vi "MKS test.vi"() -> ()   [LabVIEW 2022 SP3]
uses:
  MKS.lvclass
panel:
  out "Data":dbl[](array[numeric])
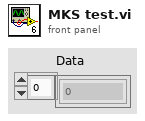
[diagram p1: front panel]
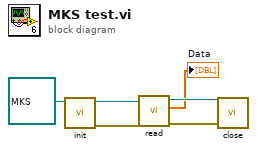
[diagram p0: block diagram]
diagram:
  n1 = call-dynamic "init.vi"("MKS in"=refnum<class "MKS.lvclass"> refnum) -> ("error out"=w2:errorcluster, "MKS out"=w6:refnum<class "MKS.lvclass">)  [unwired: 8 in, 1 out]
  n2 = call-dynamic "read.vi"("error in (no error)"=w2, "MKS in"=w6) -> ("error out"=w1:errorcluster, "Data"=→"Data":dbl[], "MKS out"=w5:refnum<class "MKS.lvclass">)  [unwired: 7 in]
  n3 = call-dynamic "close.vi"("error in (no error)"=w1, "MKS in"=w5) -> ()  [unwired: 8 in, 2 out]
